vi "Constants.vi"() -> ()   [LabVIEW 2015, in "Inline Async Example Shared.lvlib"]
doc: "Use this Global VI to access the GUIDs assigned to the page resources of the Custom Device."
uses:
  Inline Async Example Shared.lvlib
panel:
  in  "Tab Control":enum32{"GUIDS", "Constants", "Properties"}(tab)
  in  "Inline Async Example":string="d41b8ac3-b9c3-4bcd-adf6-cfb75c66b3bc"
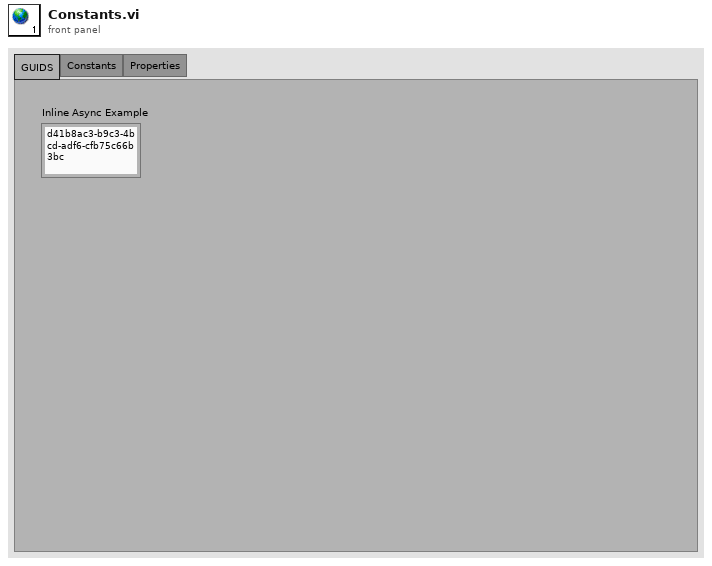
[diagram p1: front panel]
diagram:
